vi "Patch_Method.vi"(6 "Headers":cluster{"Name":string, "Value":string}[](array[cluster]), 7 "Body Content-Type":string, 8 "error in (no error)":errorcluster, 9 "Body":string, 10 "Endpoint URL":string, 11 "Request in":refnum<class "Request.lvclass">) -> (0 "error out":errorcluster, 3 "Request out":refnum<class "Request.lvclass">)   [LabVIEW 2016]
uses:
  Request.lvclass
  Response.lvclass
panel:
  out "Response out":refnum<class "Response.lvclass">
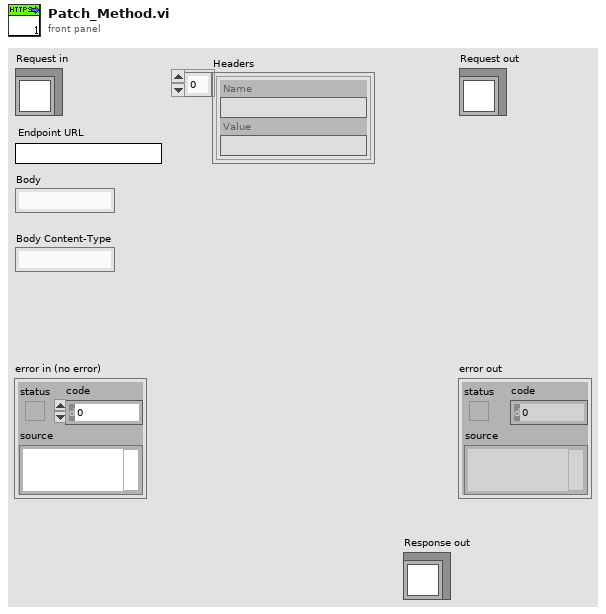
[diagram p1: front panel]
types:
  T1 = enum16{"PATCH_MULTIPART", "POST_MULTIPART", "PATCH", "DELETE", "HEAD", "PUT", "GET"}
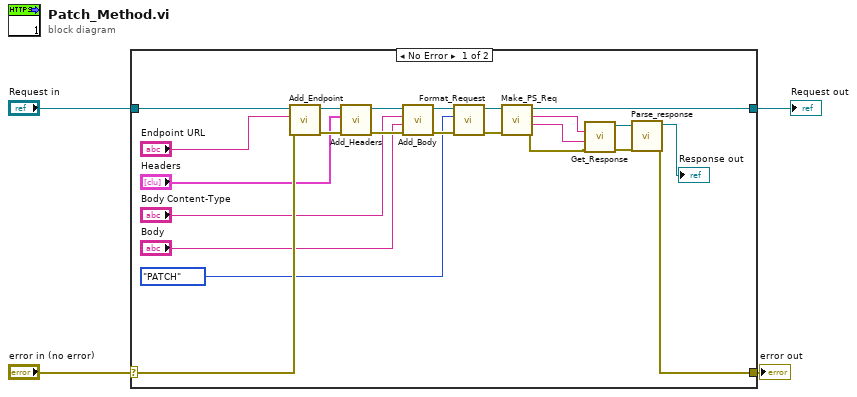
[diagram p0: block diagram]
diagram:
  n1 = case shown="No Error" "error in (no error)" {
    selector: "error in (no error)" -> [w23 w29]
    tunnel: [w11 w29] -> w3
    tunnel: [w25 w28] -> w1
    tunnel: "Request in" -> [w27 w28]
    frame No Error {
      n2 = call "Add_Endpoint.vi"("error in (no error)"=w23, "Endpoint URL"="Endpoint URL", "Request in"=w27) -> ("error out"=w24:errorcluster, "Request out"=w26:refnum<class "Request.lvclass">)  [unwired: 7 in]
      n3 = call "Add_Headers.vi"("error in (no error)"=w24, "Headers"="Headers", "Request in"=w26) -> ("error out"=w17:errorcluster, "Request out"=w18:refnum<class "Request.lvclass">)  [unwired: 7 in]
      n4 = call "Add_Body.vi"("error in (no error)"=w17, "Body"="Body", "Body Content-Type"="Body Content-Type", "Request in"=w18) -> ("error out"=w19:errorcluster, "Request out"=w20:refnum<class "Request.lvclass">)  [unwired: 6 in]
      n5 = call "Format_Request.vi"("error in (no error)"=w19, "Request"=T1."PATCH", "Request in"=w20) -> ("error out"=w22:errorcluster, "Request out"=w21:refnum<class "Request.lvclass">)  [unwired: 7 in]
      n6 = call "Make_PS_Req.vi"("error in (no error)"=w22, "Request in"=w21) -> ("error out"=w12:errorcluster, "standard error"=w5:string, "standard output"=w13:string, "Request out"=w25:refnum<class "Request.lvclass">)  [unwired: 6 in]
      n7 = call "Get_Response.vi"("error in (no error)"=w12, "PS Error"=w5, "PS Response"=w13) -> ("error out"=w15:errorcluster, "Response out"=w16:refnum<class "Response.lvclass">)  [unwired: 7 in]
      n8 = call "Parse_response.vi"("error in (no error)"=w15, "Response in"=w16) -> ("error out"=w11:errorcluster, "Response out"=→"Response out":refnum<class "Response.lvclass">)  [unwired: 8 in]
    }
    frame Error {
    }
  }
  "error out" <- w3
  "Request out" <- w1
